vi "Section2.vi"() -> ()   [LabVIEW 2023]
uses:
  Communication/PCAN2023/PCAN API.lvlib
panel:
  out "Group 2":T1
  out "Group1":T2
  out "Read NTCs":bool
  out "Enable Engine Run":bool
  out "Clear Nexteer NTCs":bool
  out "Connect2":bool
  out "Read System Status":bool
  out "Set Vehicle Speed":bool
  out "Read MEC Counter":bool
  out "Write Gain Values to default":bool
  out "Write Offset Values to default":bool
  out "Write Analog Torque Scale 5":bool
  out "Write Analog Torque Scale 4":bool
  out "Write System Friction":bool
  out "Write BEMF":bool
  out "Write Polarity":bool
  out "SW Version 2":string
  out "SW Version":bool
  out "Nexteer Connect":bool
  out "error out":errorcluster
  in  "error in":errorcluster
  in  "Channel":u16=65 format="%x"
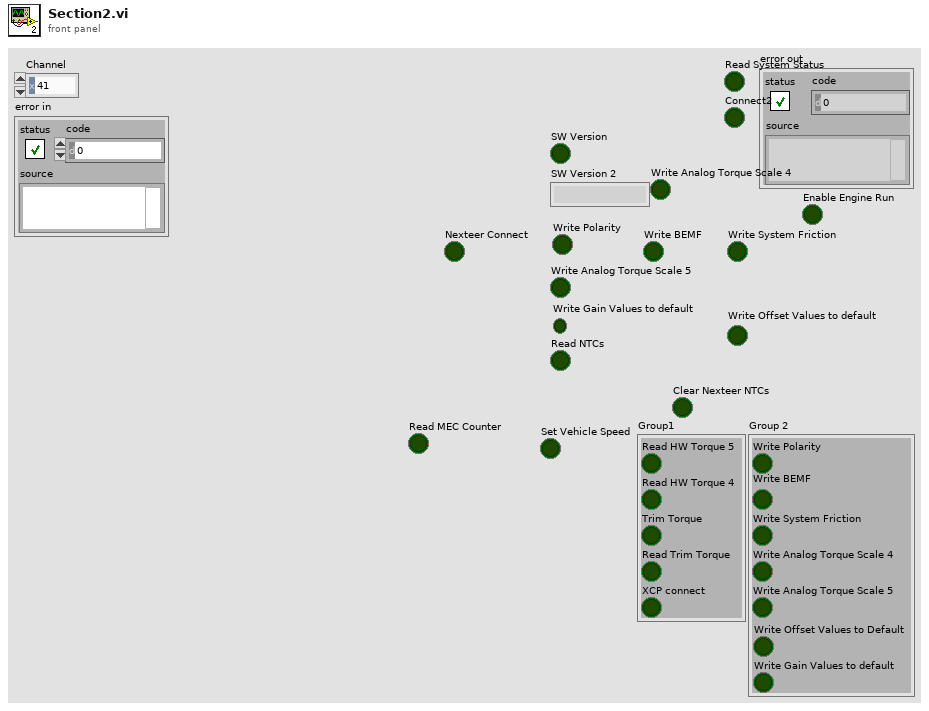
[diagram p1: front panel]
types:
  T1 = cluster{"Write Polarity":bool, "Write BEMF":bool, "Write System Friction":bool, "Write Analog Torque Scale 4":bool, "Write Analog Torque Scale 5":bool, "Write Gain Values to default":bool, "Write Offset Values to Default":bool}
  T2 = cluster{"Read HW Torque 5":bool, "Read HW Torque 4":bool, "Trim Torque":bool, "Read Trim Torque":bool, "XCP connect":bool}
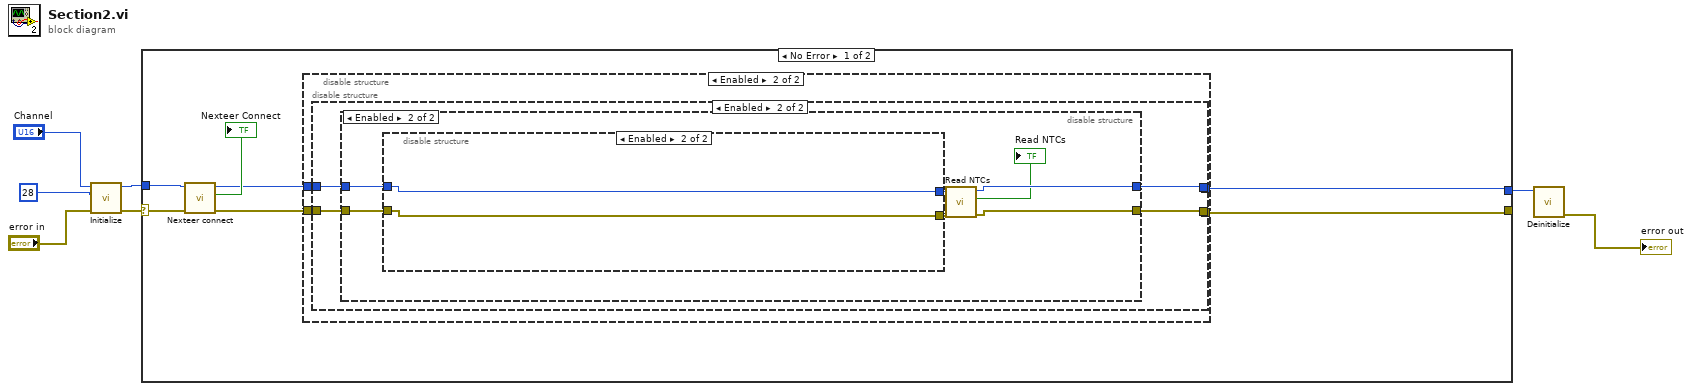
[diagram p0: block diagram]
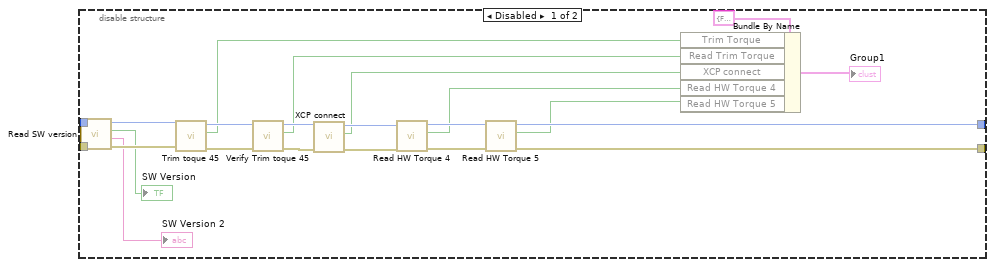
[diagram p2: hidden frame]
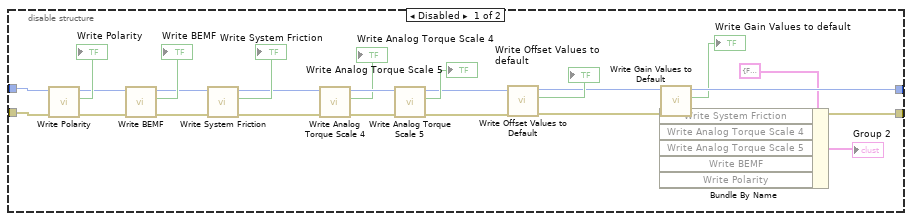
[diagram p3: hidden frame]
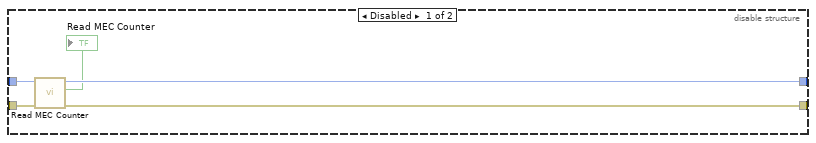
[diagram p4: hidden frame]
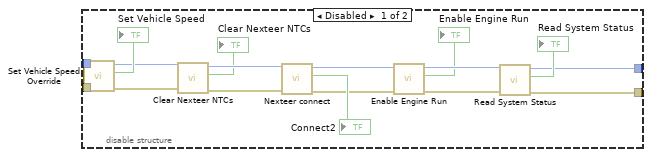
[diagram p5: hidden frame]
diagram:
  n1 = call "Initialize.vi"("error in"="error in", "Btr0Btr1"=u16 28, "Channel"="Channel") -> ("error out"=w1:errorcluster, "Channel out"=w4:u16)  [unwired: 6 in, 1 out]
  n2 = case shown="No Error" w1 {
    selector: w1 -> [w13 w104]
    tunnel: w4 -> [w14 w103]
    tunnel: [w9 w103] -> w3
    tunnel: [w8 w104] -> _
    frame No Error {
      n3 = call "Nexteer connect.vi"("error in"=w13, "Channel in"=w14) -> ("error out"=w10:errorcluster, "Pass"=→"Nexteer Connect":bool, "Channel out"=w11:u16)  [unwired: 4 in, 1 out]
      n4 = disable-structure shown="Enabled" {
        disable-tunnel: w11 -> [w31 w41]
        disable-tunnel: w10 -> [w29 w40]
        disable-tunnel: [w24 w39] -> w9
        disable-tunnel: [w22 w38] -> w8
        frame Disabled {
          n5 = call "Read SW version.vi"("error in"=w29, "Channel in"=w31) -> ("error out"=w28:errorcluster, "SW Version"=→"SW Version 2":string, "Pass"=→"SW Version":bool, "Channel out"=w30:u16)  [unwired: 4 in]
          n6 = call "Trim toque 45.vi"("error in"=w28, "Channel in"=w30) -> ("error out"=w34:errorcluster, "Pass"=w19:bool, "Channel out"=w35:u16)  [unwired: 4 in, 1 out]
          n7 = call "Verify Trim toque 45.vi"("error in"=w34, "Channel in"=w35) -> ("error out"=w36:errorcluster, "Pass"=w18:bool, "Channel out"=w37:u16)  [unwired: 4 in, 1 out]
          n8 = call "XCP connect.vi"("error in"=w36, "Channel in"=w37) -> ("error out"=w32:errorcluster, "Pass"=w17:bool, "Channel out"=w33:u16)  [unwired: 4 in, 1 out]
          n9 = call "Read HW Torque 4.vi"("error in"=w32, "Channel in"=w33) -> ("error out"=w23:errorcluster, "Pass"=w16:bool, "Channel out"=w25:u16)  [unwired: 4 in, 1 out]
          n10 = call "Read HW Torque 5.vi"("error in"=w23, "Channel in"=w25) -> ("error out"=w22:errorcluster, "Pass"=w15:bool, "Channel out"=w24:u16)  [unwired: 4 in, 1 out]
          n11 = Bundle By Name(cluster=T2 {"Read HW Torque 5"=FALSE, "Read HW Torque 4"=FALSE, "Trim Torque"=FALSE, "Read Trim Torque"=FALSE, "XCP connect"=FALSE} ("Cluster 2"), "Trim Torque"=w19, "Read Trim Torque"=w18, "XCP connect"=w17, "Read HW Torque 4"=w16, "Read HW Torque 5"=w15) -> (→"Group1":T2)
        }
        frame Enabled {
          n12 = disable-structure shown="Enabled" {
            disable-tunnel: w41 -> [w67 w71]
            disable-tunnel: w40 -> [w66 w70]
            disable-tunnel: [w48 w69] -> w39
            disable-tunnel: [w46 w68] -> w38
            frame Disabled {
              n13 = call "Write Polarity.vi"("error in"=w66, "Channel in"=w67) -> ("error out"=w63:errorcluster, "Pass"=→"Write Polarity":bool, "Channel out"=w64:u16)  [unwired: 4 in, 1 out]
              n14 = call "Write BEMF.vi"("error in"=w63, "Channel in"=w64) -> ("error out"=w60:errorcluster, "Pass"=→"Write BEMF":bool, "Channel out"=w61:u16)  [unwired: 4 in, 1 out]
              n15 = call "Write System Friction.vi"("error in"=w60, "Channel in"=w61) -> ("error out"=w56:errorcluster, "Pass"=→"Write System Friction":bool, "Channel out"=w58:u16)  [unwired: 4 in, 1 out]
              n16 = call "Write Analog Torque Scale 4.vi"("error in"=w56, "Channel in"=w58) -> ("error out"=w55:errorcluster, "Pass"=→"Write Analog Torque Scale 4":bool, "Channel out"=w57:u16)  [unwired: 4 in, 1 out]
              n17 = call "Write Analog Torque Scale 5.vi"("error in"=w55, "Channel in"=w57) -> ("error out"=w51:errorcluster, "Pass"=→"Write Analog Torque Scale 5":bool, "Channel out"=w52:u16)  [unwired: 4 in, 1 out]
              n18 = call "Write Offset Values to Default.vi"("error in"=w51, "Channel in"=w52) -> ("error out"=w47:errorcluster, "Pass"=→"Write Offset Values to default":bool, "Channel out"=w49:u16)  [unwired: 4 in, 1 out]
              n19 = Bundle By Name(cluster=T1 {"Write Polarity"=FALSE, "Write BEMF"=FALSE, "Write System Friction"=FALSE, "Write Analog Torque Scale 4"=FALSE, "Write Analog Torque Scale 5"=FALSE, "Write Gain Values to default"=FALSE, "Write Offset Values to Default"=FALSE} ("Group 2")) -> (→"Group 2":T1, "Write Polarity"=w44:bool)  [unwired: 4 in]
              n20 = call "Write Gain Values to Default.vi"("error in"=w47, "Channel in"=w49) -> ("error out"=w46:errorcluster, "Pass"=→"Write Gain Values to default":bool, "Channel out"=w48:u16)  [unwired: 4 in, 1 out]
            }
            frame Enabled {
              n21 = disable-structure shown="Enabled" {
                disable-tunnel: w71 -> [w76 w83]
                disable-tunnel: w70 -> [w75 w82]
                disable-tunnel: [w74 w80] -> w69
                disable-tunnel: [w73 w78] -> w68
                frame Disabled {
                  n22 = call "Read MEC Counter.vi"("error in"=w75, "Channel in"=w76) -> ("error out"=w73:errorcluster, "Pass"=→"Read MEC Counter":bool, "Channel out"=w74:u16)  [unwired: 4 in, 1 out]
                }
                frame Enabled {
                  n23 = disable-structure shown="Enabled" {
                    disable-tunnel: w83 -> [w100 w102]
                    disable-tunnel: w82 -> [w99 w101]
                    disable-tunnel: [w85 w102] -> w81
                    disable-tunnel: [w84 w101] -> w79
                    frame Disabled {
                      n24 = call "Set Vehicle Speed Override.vi"("error in"=w99, "Channel in"=w100) -> ("error out"=w93:errorcluster, "Pass"=→"Set Vehicle Speed":bool, "Channel out"=w95:u16)  [unwired: 4 in, 1 out]
                      n25 = call "Clear Nexteer NTCs.vi"("error in"=w93, "Channel in"=w95) -> ("error out"=w92:errorcluster, "Pass"=→"Clear Nexteer NTCs":bool, "Channel out"=w94:u16)  [unwired: 4 in, 1 out]
                      n26 = call "Nexteer connect.vi"("error in"=w92, "Channel in"=w94) -> ("error out"=w88:errorcluster, "Pass"=→"Connect2":bool, "Channel out"=w90:u16)  [unwired: 4 in, 1 out]
                      n27 = call "Enable Engine Run.vi"("error in"=w88, "Channel in"=w90) -> ("error out"=w87:errorcluster, "Pass"=→"Enable Engine Run":bool, "Channel out"=w89:u16)  [unwired: 4 in, 1 out]
                      n28 = call "Read System Status.vi"("error in"=w87, "Channel in"=w89) -> ("error out"=w84:errorcluster, "Pass"=→"Read System Status":bool, "Channel out"=w85:u16)  [unwired: 4 in, 1 out]
                    }
                    frame Enabled {
                    }
                  }
                  n29 = call "Read NTCs.vi"("error in"=w79, "Channel in"=w81) -> ("error out"=w78:errorcluster, "Pass"=→"Read NTCs":bool, "Channel out"=w80:u16)  [unwired: 5 in]
                }
              }
            }
          }
        }
      }
    }
    frame Error {
    }
  }
  n30 = call "Deinitialize.vi"("Channel"=w3) -> ("error out"=→"error out":errorcluster)  [unwired: 10 in]
